vi "Set t0.vi"(10 "T0":timestamp, 11 "WavBuf":refnum<class "WavBuf.lvclass">) -> (3 "WavBuf Out":refnum<class "WavBuf.lvclass">)   [LabVIEW 2020, in "WavBuf.lvclass"]
uses:
  WavBuf.lvclass
  WavBuf.lvclass/WavBuf.ctl
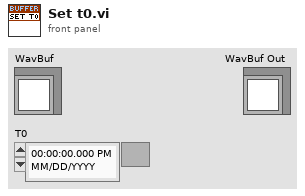
[diagram p1: front panel]
types:
  T1 = typedef "Ref_DVR_Buffer.ctl" = refnum<data-value>
  T2 = typedef "Waveform_Data.ctl" = waveform(dbl)
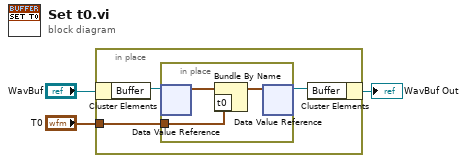
[diagram p0: block diagram]
diagram:
  n1 = in-place {
    in-place-border: "T0" -> [w6]
    n2 = in-place-cluster #1("WavBuf") -> ("Buffer"=w5:T1)
    n3 = in-place {
      in-place-border: w6 -> [w7]
      n4 = in-place-dvr #2(w5) -> (w9:T2)  [unwired: 1 out]
      n5 = Bundle By Name(cluster=w9, "t0"=w7) -> (w8:T2)
      n6 = in-place-dvr #2(w8) -> (w4:T1)  [unwired: 1 out]
    }
    n7 = in-place-cluster #1("Buffer"=w4) -> (→"WavBuf Out":refnum<class "WavBuf.lvclass">)
  }
